vi "Average_Time_array.vi"(2 "Average TIme (seconds)":dbl, 3 "Centre Time in Seconds":dbl[](array[numeric])) -> (0 "Length":i32[](array[numeric]), 1 "Start":i32[](array[numeric]))   [LabVIEW 2010]
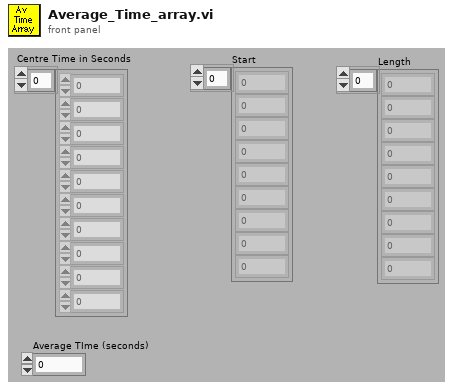
[diagram p1: front panel]
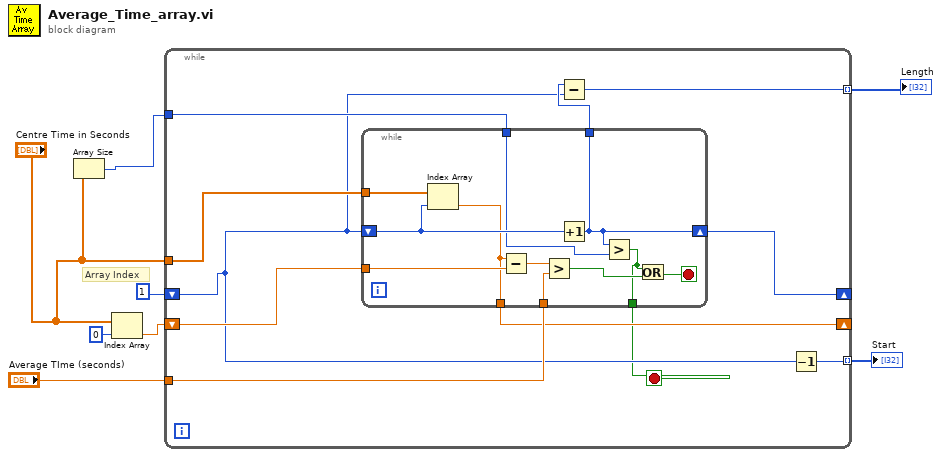
[diagram p0: block diagram]
diagram:
  # "Array Index"
  n1 = Array Size(array="Centre Time in Seconds") -> (size(s)=w1:i32)
  n2 = Index Array(array="Centre Time in Seconds", index=0) -> (element=w6:dbl)
  n3 = while {
    shift-right: [w15] -> _
    shift-left: 1 -> [w11]
    shift-right: [w14] -> _
    shift-left: w6 -> [w18]
    tunnel: "Centre Time in Seconds" -> [w19]
    tunnel: "Average TIme (seconds)" -> [w17]
    tunnel: w1 -> [w16]
    tunnel: [w12] -> w3 mode=indexing
    tunnel: [w10] -> w2 mode=indexing
    stop <- w9 stop-if-true
    n4 = while {
      shift-right: [w20] -> w15
      shift-left: w11 -> [w29]
      tunnel: w19 -> [w30]
      tunnel: w18 -> [w27]
      tunnel: w17 -> [w26]
      tunnel: w16 -> [w25]
      tunnel: [w22] -> w9
      tunnel: [w21] -> w14
      tunnel: [w20] -> w13
      stop <- w23 stop-if-true
      n5 = Index Array(array=w30, index=w29) -> (element=w21:dbl)
      n6 = Subtract(x=w21, y=w27) -> (x-y=w28:dbl)
      n7 = Greater?(x=w28, y=w26) -> (0:w24:bool)
      n8 = Increment(x=w29) -> (x+1=w20:i32)
      n9 = Greater?(x=w20, y=w25) -> (0:w22:bool)
      n10 = Or(x=w22, y=w24) -> (x .or. y?=w23:bool)
    }
    n11 = Subtract(x=w13, y=w11) -> (x-y=w12:i32)
    n12 = Decrement(x=w11) -> (x-1=w10:i32)
  }
  "Length" <- w3
  "Start" <- w2
